vi "Format Measurement Parameters.vi"(8 "error in (no error)":errorcluster, 10 "Measurement Parameters In":refnum<class "String Database.lvclass">[](array[class]), 11 "QPA TCF Parser in":refnum<class "QPA TCF Parser.lvclass">) -> (0 "error out":errorcluster, 2 "Measurement Parameters Out":refnum<class "String Database.lvclass">[](array[class]), 3 "QPA TCF Parser out":refnum<class "QPA TCF Parser.lvclass">)   [LabVIEW 2016, in "QPA TCF Parser.lvlib" / "QPA TCF Parser.lvclass"]
uses:
  QPA TCF Parser.lvclass
  Plugins/String Database.lvlibp/String Database.lvclass
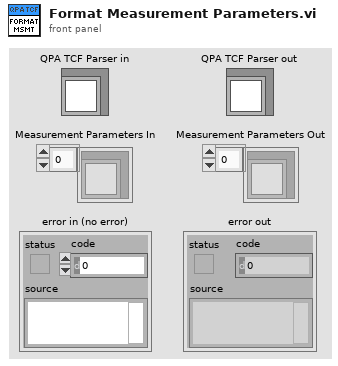
[diagram p1: front panel]
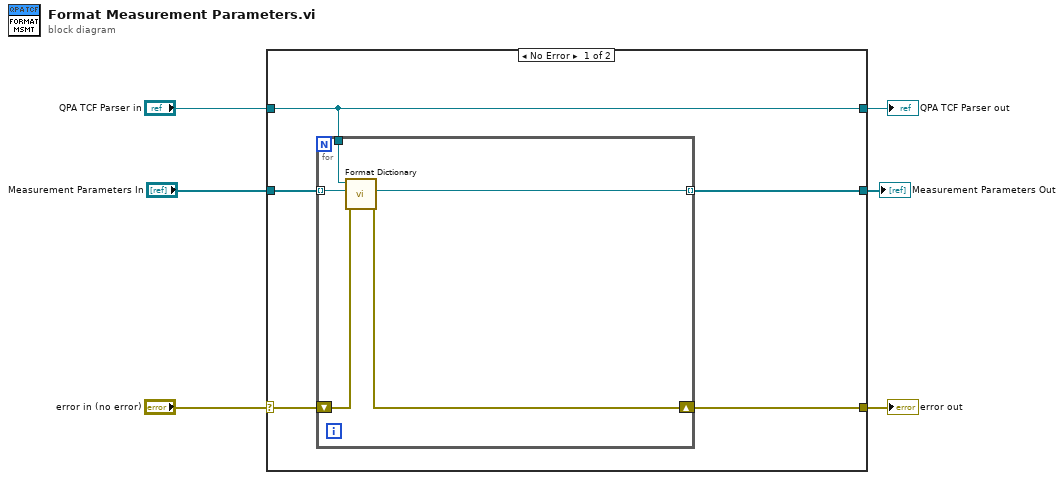
[diagram p0: block diagram]
diagram:
  n1 = case shown="No Error" "error in (no error)" {
    selector: "error in (no error)" -> [w9 w19]
    tunnel: [w8 w19] -> w5
    tunnel: [w10 w18] -> w3
    tunnel: "QPA TCF Parser in" -> [w10 w18]
    tunnel: [w7 w17] -> w2
    tunnel: "Measurement Parameters In" -> [w11 w17]
    frame No Error {
      n2 = for {
        tunnel: w11 -> [w15] mode=indexing
        tunnel: w10 -> [w13]
        shift-right: [w12] -> w8
        shift-left: w9 -> [w16]
        tunnel: [w14] -> w7 mode=indexing
        n3 = call "Format Dictionary.vi"("error in (no error)"=w16, "Measurement Parameters In"=w15, "QPA TCF Parser in"=w13) -> ("error out"=w12:errorcluster, "String Database out"=w14:refnum<class "String Database.lvclass">)  [unwired: 6 in]
      }
    }
    frame Error {
    }
  }
  "error out" <- w5
  "QPA TCF Parser out" <- w3
  "Measurement Parameters Out" <- w2
